vi "Read_IMU_9dof.vi"() -> ()   [LabVIEW 2018]
uses:
  <vilib>/Instr/_visa.llb/VISA Configure Serial Port (Instr).vi
  <vilib>/regexp/Match Regular Expression.xnode
panel:
  in  "Stop":bool
  out "Euler Angles":cluster{"Pitch":dbl, "Roll":dbl, "Yaw":dbl}
  in  "Serial Settings":T1={"baud rate"=9600, "data bits"=8, "parity"=enum."None", "stop bits"=10, "flow control"=1} {"flow control" items=["None"=0, "XON/XOFF"=1, "RTS/CTS"=2, "DTR/DSR"=4]; "stop bits" items=["1.0"=10, "1.5"=15, "2.0"=20]; "data bits" min=5 max=8 step=1; "baud rate" items=["75"=75, "110"=110, "134"=134, "150"=150, "300"=300, "600"=600, "1200"=1200, "1800"=1800, "2400"=2400, "4800"=4800, "7200"=7200, "9600"=9600, "14400"=14400, "19200"=19200, "28800"=28800, "38400"=38400, "56000"=56000, "57600"=57600, "115200"=115200, "128000"=128000, "230400"=230400]}
  in  "VISA resource name":refnum<visa-resource-name>="COM5"
  in  "Termination Character":u8=10 format="%.0x"
  in  "XON/XOFF Characters":T2={"XON"=enum."DC1", "XOFF"=enum."DC3"}
  in  "Termination Character?":bool=TRUE
  in  "Read Count":u32=1000
  # "COM Port"
  # "COM Setings"
  # "COM Specific"
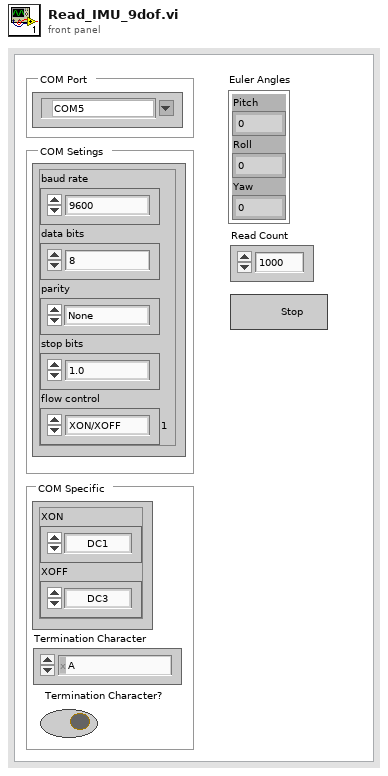
[diagram p1: front panel]
types:
  T1 = cluster{"baud rate":u32, "data bits":u16, "parity":enum16{"None", "Odd", "Even", "Mark", "Space"}, "stop bits":u16, "flow control":u16}
  T2 = cluster{"XON":enum16{"NUL", "SOH", "STX", "ETX", "EOT", "ENQ", "ACK", "BEL", "BS", "HT", "LF", "VT", "FF", "CR", "SO", "SI", "DLE", "DC1", "DC2", "DC3", "DC4", "NAK", "SYN", "ETB", "CAN", "EM", "SUB", "ESC", "FS", "GS", "RS", "US", "SP", "!", "\"", "#", "$", "%", "&", "'", "(", ")", "*", "+", ",", "- (-)", ".", "/", "0", "1", "2", "3", "4", "5", "6", "7", "8", "9", ":", ";", "<", "=", ">", "?", "@", "A", "B", "C", "D", "E", "F", "G", "H", "I", "J", "K", "L", "M", "N", "O", "P", "Q", "R", "S", "T", "U", "V", "W", "X", "Y", "Z", "[", "\\", "]", "^", "_", "`", "a", "b", "c", "d", "e", "f", "g", "h", "i", "j", "k", "l", "m", "n", "o", "p", "q", "r", "s", "t", "u", "v", "w", "x", "y", "z", "{", "|", "}", "~"}, "XOFF":enum16{"NUL", "SOH", "STX", "ETX", "EOT", "ENQ", "ACK", "BEL", "BS", "HT", "LF", "VT", "FF", "CR", "SO", "SI", "DLE", "DC1", "DC2", "DC3", "DC4", "NAK", "SYN", "ETB", "CAN", "EM", "SUB", "ESC", "FS", "GS", "RS", "US", "SP", "!", "\"", "#", "$", "%", "&", "'", "(", ")", "*", "+", ",", "- (-)", ".", "/", "0", "1", "2", "3", "4", "5", "6", "7", "8", "9", ":", ";", "<", "=", ">", "?", "@", "A", "B", "C", "D", "E", "F", "G", "H", "I", "J", "K", "L", "M", "N", "O", "P", "Q", "R", "S", "T", "U", "V", "W", "X", "Y", "Z", "[", "\\", "]", "^", "_", "`", "a", "b", "c", "d", "e", "f", "g", "h", "i", "j", "k", "l", "m", "n", "o", "p", "q", "r", "s", "t", "u", "v", "w", "x", "y", "z", "{", "|", "}", "~"}}
  T3 = enum16{"NUL", "SOH", "STX", "ETX", "EOT", "ENQ", "ACK", "BEL", "BS", "HT", "LF", "VT", "FF", "CR", "SO", "SI", "DLE", "DC1", "DC2", "DC3", "DC4", "NAK", "SYN", "ETB", "CAN", "EM", "SUB", "ESC", "FS", "GS", "RS", "US", "SP", "!", "\"", "#", "$", "%", "&", "'", "(", ")", "*", "+", ",", "- (-)", ".", "/", "0", "1", "2", "3", "4", "5", "6", "7", "8", "9", ":", ";", "<", "=", ">", "?", "@", "A", "B", "C", "D", "E", "F", "G", "H", "I", "J", "K", "L", "M", "N", "O", "P", "Q", "R", "S", "T", "U", "V", "W", "X", "Y", "Z", "[", "\\", "]", "^", "_", "`", "a", "b", "c", "d", "e", "f", "g", "h", "i", "j", "k", "l", "m", "n", "o", "p", "q", "r", "s", "t", "u", "v", "w", "x", "y", "z", "{", "|", "}", "~"}
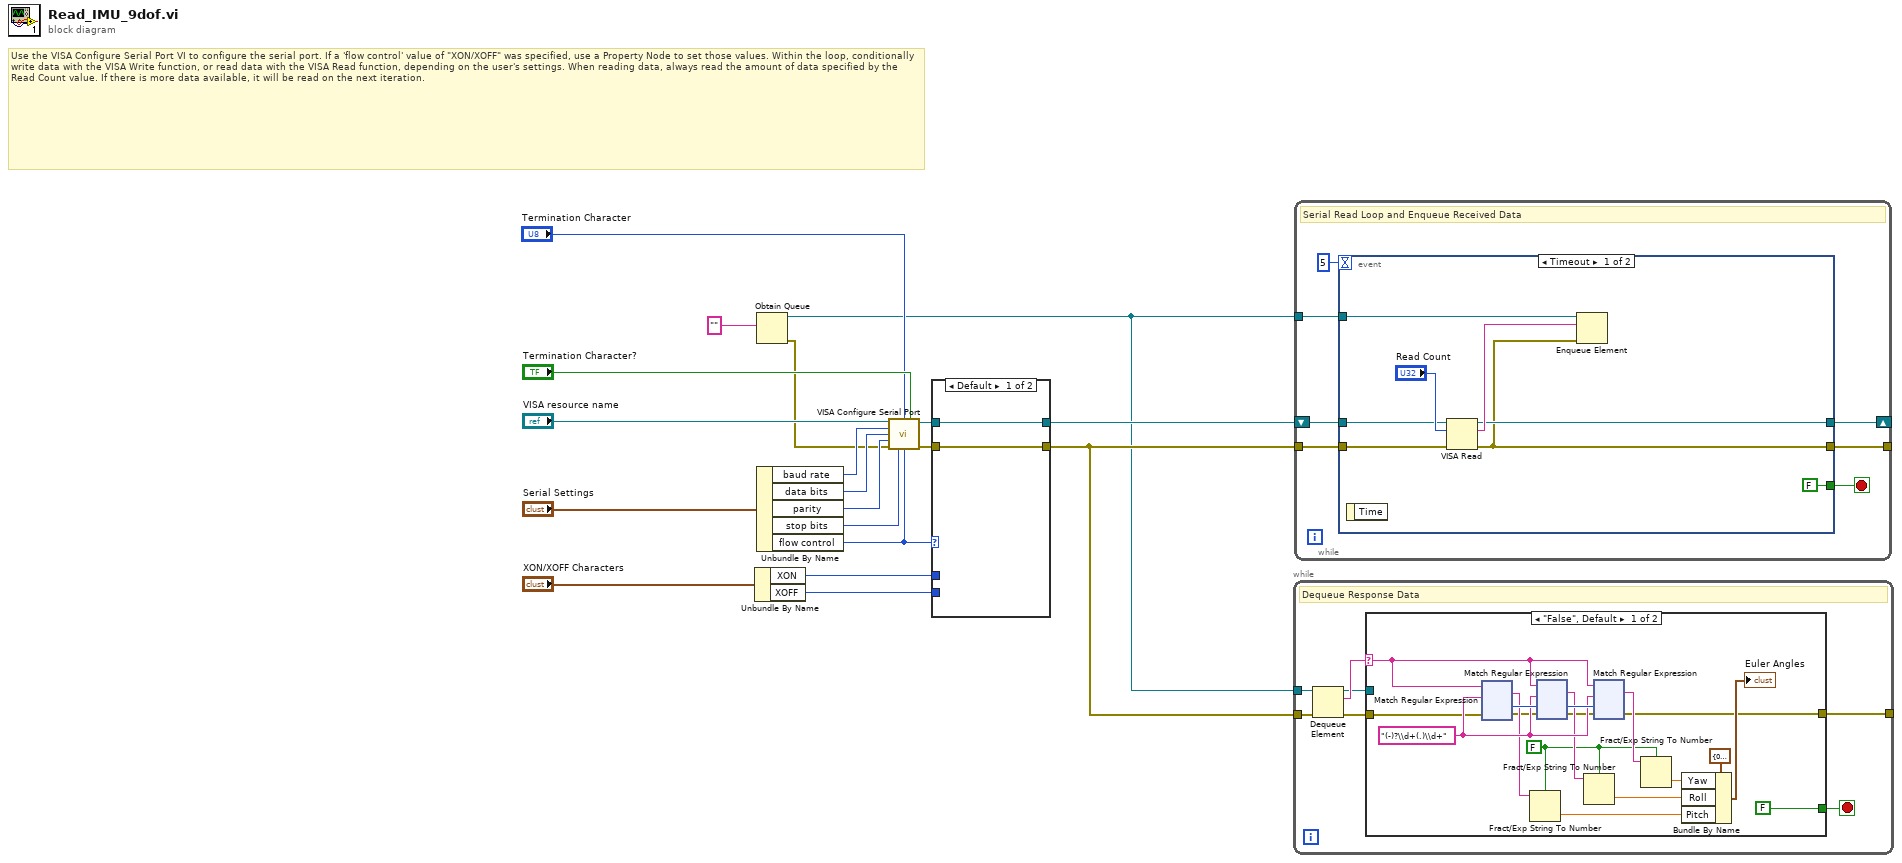
[diagram p0: block diagram]
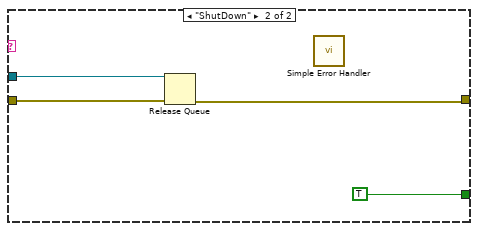
[diagram p2: hidden frame]
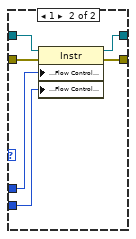
[diagram p3: hidden frame]
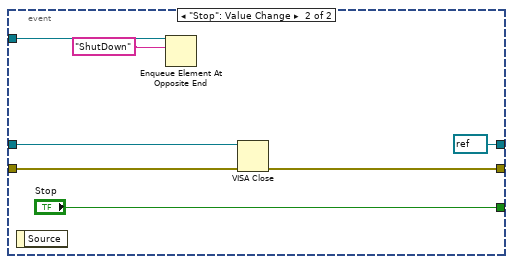
[diagram p4: hidden frame]
diagram:
  # "Use the VISA Configure Serial Port VI to configure the serial port. If a 'flow control' value of \"XON/XOFF\" was specified, use a Property Node to set those values. Within the loop, conditionally write data with the VISA Write function, or read data with the VISA Read function, depending on the user's settings. When reading data, always read the amount of data specified by the Read Count value. If there is more data available, it will be read on the next iteration."
  n1 = Unbundle By Name("XON/XOFF Characters") -> ("XON"=w8:T3, "XOFF"=w7:T3)
  n2 = Obtain Queue(element data type="" ("read buffer")) -> (queue out=w1:refnum<queue>, error out=w5:errorcluster)  [unwired: 4 in, 1 out]
  n3 = Unbundle By Name("Serial Settings") -> ("baud rate"=w12:u32, "data bits"=w13:u16, "parity"=w14:enum16{"None", "Odd", "Even", "Mark", "Space"}, "stop bits"=w15:u16, "flow control"=w9:u16)
  n4 = call-poly "VISA Configure Serial Port"("VISA resource name"="VISA resource name", "termination char\n(0xA = '\\n' = LF)"="Termination Character", "Enable Termination\nChar (T)"="Termination Character?", "baud rate (9600)"=w12, "data bits (8)"=w13, "parity (0:none)"=w14, "error in (no error)"=w5, "stop bits (10: 1 bit)"=w15, "flow control (0:none)"=w9) -> ("VISA resource name out"=w16:refnum<visa-resource-name>, "error out"=w17:errorcluster)  [unwired: 1 in, 4 out]
  n5 = case shown="Default" w9 {
    tunnel: [w20 w27] -> w3
    tunnel: [w21 w26] -> w2
    tunnel: w17 -> [w20 w25]
    tunnel: w16 -> [w21 w24]
    tunnel: w8 -> [_ w23]
    tunnel: w7 -> [_ w22]
    frame Default {
    }
    frame 1 {
      n6 = property class="Instr"(reference=w24, error in=w25, "Serial Settings:Flow Control XON Character"=w23, "Serial Settings:Flow Control XOFF Character"=w22) -> (reference out=w26:refnum<visa-resource-name>, error out=w27:errorcluster)
    }
  }
  n7 = while {
    tunnel: w1 -> [w34]
    tunnel: w3 -> [w33]
    tunnel: [w28] -> _
    stop <- w29 stop-if-true
    # "Dequeue Response Data"
    n8 = Dequeue Element(queue=w34, error in (no error)=w33) -> (queue out=w31:refnum<queue>, element=w32:string, error out=w30:errorcluster)  [unwired: 1 in, 1 out]
    n9 = case shown="\"False\", Default" w32 {
      selector: w32 -> [w39 _]
      tunnel: w31 -> [_ w398]
      tunnel: w30 -> [w38 w397]
      tunnel: [FALSE TRUE] -> w29
      tunnel: [w35 w395] -> w28
      frame "False", Default {
        w45 = FALSE ("use system decimal point (T)")
        w49 = "(-)?\\d+(.)\\d+" ("regular expression")
        n10 = xnode "Match Regular Expression"("input string"=w39, "regular expression"=w49, "error in"=w38) -> ("whole match"=w48:string, "offset past match"=w51:i32, "error out"=w37:errorcluster)  [unwired: 3 in, 2 out]
        n11 = Fract/Exp String To Number(use system decimal point (T)=w45, string=w48) -> (number=w41:dbl)  [unwired: 2 in, 1 out]
        n12 = xnode "Match Regular Expression"("input string"=w39, "regular expression"=w49, "offset (0)"=w51, "error in"=w37) -> ("whole match"=w47:string, "offset past match"=w50:i32, "error out"=w36:errorcluster)  [unwired: 2 in, 2 out]
        n13 = Fract/Exp String To Number(use system decimal point (T)=w45, string=w47) -> (number=w42:dbl)  [unwired: 2 in, 1 out]
        n14 = xnode "Match Regular Expression"("input string"=w39, "regular expression"=w49, "offset (0)"=w50, "error in"=w36) -> ("whole match"=w46:string, "error out"=w35:errorcluster)  [unwired: 2 in, 3 out]
        n15 = Fract/Exp String To Number(use system decimal point (T)=w45, string=w46) -> (number=w43:dbl)  [unwired: 2 in, 1 out]
        n16 = Bundle By Name(cluster=cluster{"Pitch":dbl, "Roll":dbl, "Yaw":dbl} {"Pitch"=0.0, "Roll"=0.0, "Yaw"=0.0} ("Euler Angles"), "Yaw"=w43, "Roll"=w42, "Pitch"=w41) -> (→"Euler Angles":cluster{"Pitch":dbl, "Roll":dbl, "Yaw":dbl})
      }
      frame "ShutDown" {
        n17 = Release Queue(queue=w398, error in (no error)=w397) -> (error out=w395:errorcluster)  [unwired: 1 in, 2 out]
        n18 = call <vilib>:"Simple Error Handler.vi"() -> ()  [unwired: 2 in, 8 out]
      }
    }
  }
  n19 = while {
    shift-right: [w401] -> _
    shift-left: w2 -> [w404]
    tunnel: w3 -> [w403]
    tunnel: w1 -> [w405]
    tunnel: [w399] -> _
    stop <- w400 stop-if-true
    # "Serial Read Loop and Enqueue Received Data"
    n20 = event shown="[0] Timeout" {
      selector: _ -> [_ _]
      dyn-events: _ -> [_ _]
      timeout: 5 -> [_ _]
      tunnel: [FALSE ("Stop") "Stop"] -> w400
      tunnel: w405 -> [w408 w419]
      tunnel: w404 -> [w411 w417]
      tunnel: w403 -> [w410 w415]
      tunnel: [w409 refnum<visa-resource-name> refnum ("VISA resource name out")] -> w401
      tunnel: [w406 w414] -> w399
      event Timeout {
        n21 = event-data() -> ()  [unwired: 1 in, 1 out]
        n22 = VISA Read(VISA resource name=w411, byte count="Read Count", error in (no error)=w410) -> (VISA resource name out=w409:refnum<visa-resource-name>, read buffer=w412:string, error out=w406:errorcluster)  [unwired: 1 out]
        n23 = Enqueue Element(queue=w408, element=w412, error in (no error)=w406) -> ()  [unwired: 1 in, 3 out]
      }
      event "Stop": Value Change {
        n24 = event-data() -> ()  [unwired: 1 in, 1 out]
        n25 = Enqueue Element At Opposite End(queue=w419, element="ShutDown") -> ()  [unwired: 2 in, 3 out]
        n26 = VISA Close(VISA resource name=w417, error in (no error)=w415) -> (error out=w414:errorcluster)
      }
    }
  }
